vi "SPI_READ.vi"(11 "cluster in":cluster{bool, bool, bool}[](array[cluster])) -> (0 "IndxReadData":i32[](array[numeric]), 3 "cluster out":cluster{bool, bool, bool}[](array[cluster]), 4 "size(s)":i32)   [LabVIEW 2018]
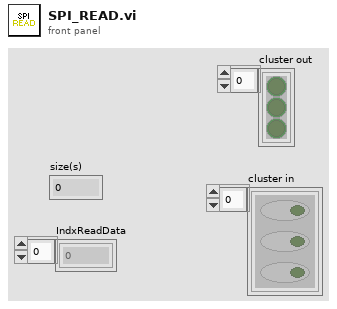
[diagram p1: front panel]
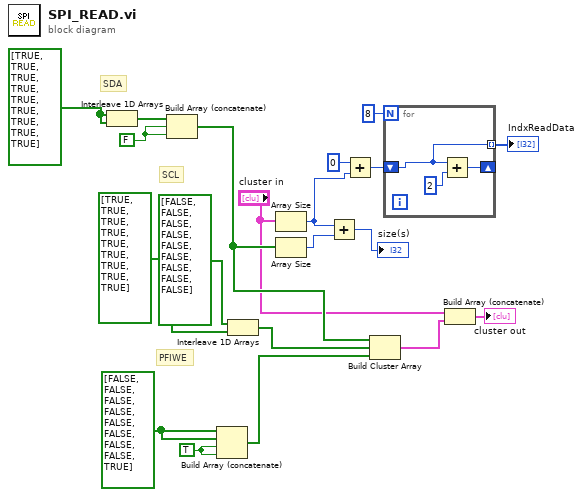
[diagram p0: block diagram]
diagram:
  w12 = bool[] [TRUE, TRUE, TRUE, TRUE, TRUE, TRUE, TRUE, TRUE, TRUE]
  w19 = TRUE
  w20 = FALSE
  w16 = bool[] [FALSE, FALSE, FALSE, FALSE, FALSE, FALSE, FALSE, FALSE, TRUE]
  # "PFIWE"
  # "SCL"
  # "SDA"
  n1 = Interleave 1D Arrays(w12, w12) -> (w15:bool[])
  n2 = Build Array (concatenate)(w15, w20, w20) -> (w6:bool[])
  n3 = Build Array (concatenate)(w16, w16, w19, w19) -> (w5:bool[])
  n4 = Interleave 1D Arrays(bool[] [FALSE, FALSE, FALSE, FALSE, FALSE, FALSE, FALSE, FALSE, FALSE], bool[] [TRUE, TRUE, TRUE, TRUE, TRUE, TRUE, TRUE, TRUE, TRUE]) -> (w7:bool[])
  n5 = Array Size(array="cluster in") -> (size(s)=w2:i32)
  n6 = Array Size(array=w6) -> (size(s)=w13:i32)
  n7 = Add(x=w2, y=w13) -> (x+y=→"size(s)":i32)
  n8 = Add(x=0, y=w2) -> (x+y=w10:i32)
  n9 = Build Cluster Array(w6, w7, w5) -> (w4:cluster{bool, bool, bool}[])
  n10 = for {
    N: 8 -> [_]
    shift-right: [w23] -> _
    shift-left: w10 -> [w21]
    tunnel: [w21] -> w9 mode=indexing
    n11 = Add(x=w21, y=2) -> (x+y=w23:i32)
  }
  "IndxReadData" <- w9
  n12 = Build Array (concatenate)("cluster in", w4) -> (→"cluster out":cluster{bool, bool, bool}[])
